vi "DataXML showXMLString.vi"(8 "error in (no error)":errorcluster, 11 "DataXML in":refnum<class "DataXML.lvclass">) -> (0 "error out":errorcluster, 1 "XML":string, 2 "Array":string[](array[string]), 3 "DataXML out":refnum<class "DataXML.lvclass">)   [LabVIEW 2018, in "DataXML.lvclass"]
uses:
  DataXML.lvclass
  DataXML.lvclass/DataXML.ctl
  <resource>/objmgr/DOMUserDefRef.rc
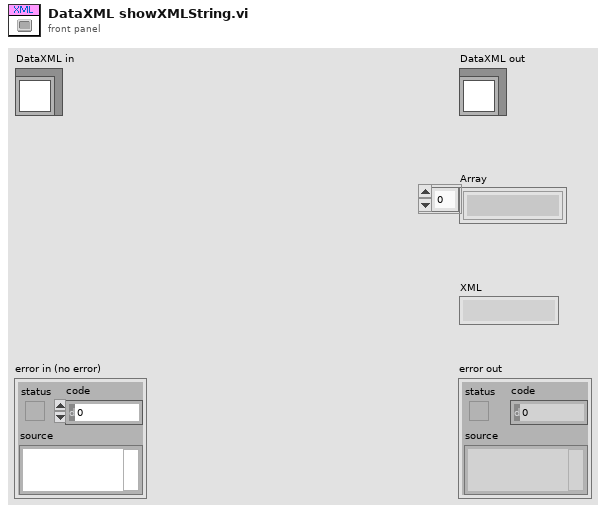
[diagram p1: front panel]
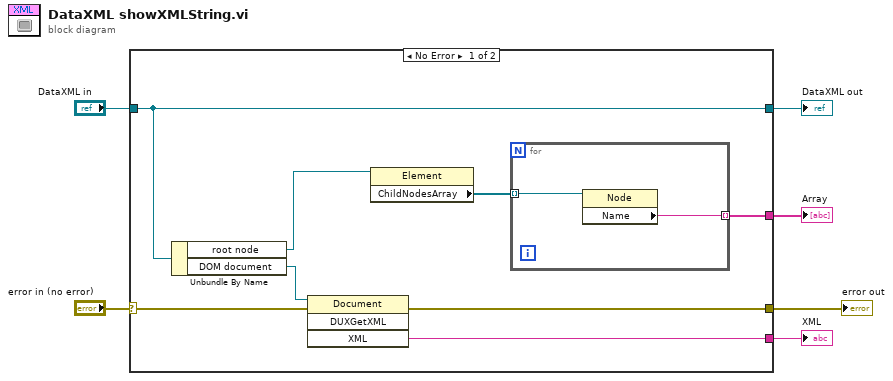
[diagram p0: block diagram]
diagram:
  n1 = case shown="No Error" "error in (no error)" {
    selector: "error in (no error)" -> [w12 w18]
    tunnel: [w11 w18] -> w5
    tunnel: [w14 w17] -> w3
    tunnel: "DataXML in" -> [w14 w17]
    tunnel: [w10 _] -> w2
    tunnel: [w7 _] -> w1
    frame No Error {
      n2 = Unbundle By Name(w14) -> ("root node"=w9:refnum<k20>, "DOM document"=w13:refnum<k20>)
      n3 = invoke class="Document" method="DUXGetXML"(reference=w13, error in=w12) -> (error out=w11:errorcluster, "XML"=w10:string)  [unwired: 2 in, 2 out]
      n4 = property class="Element"(reference=w9) -> ("ChildNodesArray"=w8:refnum<k20>[])  [unwired: 1 in, 2 out]
      n5 = for {
        tunnel: w8 -> [w16] mode=indexing
        tunnel: [w15] -> w7 mode=indexing
        n6 = property class="Node"(reference=w16) -> ("Name"=w15:string)  [unwired: 1 in, 2 out]
      }
    }
    frame Error {
    }
  }
  "error out" <- w5
  "DataXML out" <- w3
  "XML" <- w2
  "Array" <- w1
